vi "Get Log File Additional Properties.vi"(8 "error in":errorcluster, 11 "log file in":T1 format="%.0x") -> (0 "error out":errorcluster, 1 "property values":string[](array[string]), 2 "property names":string[](array[string]), 3 "log file out":T1 format="%.0x")   [LabVIEW 2027, in "Embedded Data Logger Scripting.lvlib"]
uses:
  Embedded Data Logger Scripting.lvlib
  <vilib>/NI VeriStand/Custom Device API/Custom Device Item Ref.ctl
  Shared/Constants.vi
  <vilib>/NI VeriStand/Custom Device API/Get Item Property (String Array).vi
  Shared/Embedded Data Logger Shared.lvlib
  <vilib>/NI VeriStand/Custom Device API/Custom Device API.lvlib
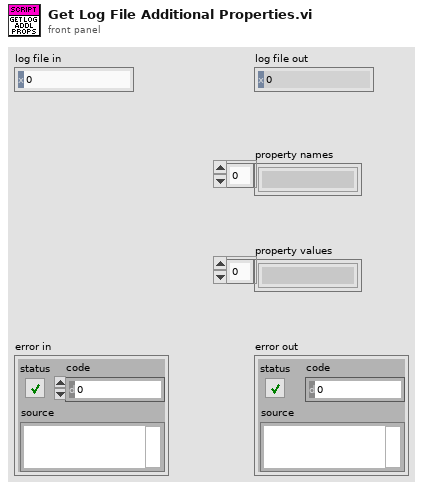
[diagram p1: front panel]
types:
  T1 = typedef "Custom Device API.lvlib/Custom Device Item Ref.ctl" = u64
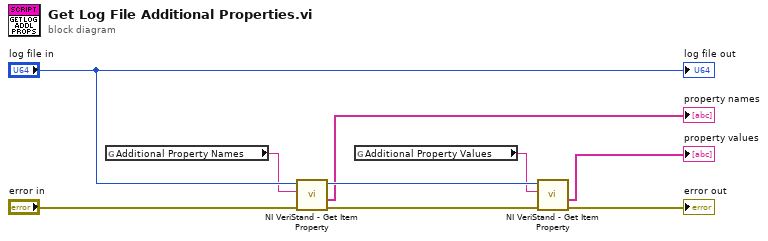
[diagram p0: block diagram]
diagram:
  n1 = global read "Constants.vi" "Additional Property Names"() -> (w6:string)
  n2 = call-poly <vilib>:"NI VeriStand - Get Item Property.vi"("error in (no error)"="error in", "Property Name"=w6, "Item Ref in"="log file in") -> ("error out"=w5:errorcluster, "Value"=→"property names":string[], "Item Ref out"=w4:T1)  [unwired: 5 in, 1 out]
  n3 = global read "Constants.vi" "Additional Property Values"() -> (w3:string)
  n4 = call-poly <vilib>:"NI VeriStand - Get Item Property.vi"("error in (no error)"=w5, "Property Name"=w3, "Item Ref in"=w4) -> ("error out"=→"error out":errorcluster, "Value"=→"property values":string[])  [unwired: 5 in, 2 out]
  "log file out" <- "log file in"
